vi "Read Value.vi"(8 "error in (no error)":errorcluster caption="entrée d'erreur (pas d'erreur)", 11 "DAQmxTaskDInput_Emulate en entrée":refnum<class "DAQmxTaskDInput_Emulate.lvclass">) -> (0 "error out":errorcluster caption="sortie d'erreur", 1 "Data":bool, 2 "Data string":string, 3 "DAQmxTaskDInput_Emulate en sortie":refnum<class "DAQmxTaskDInput_Emulate.lvclass">)   [LabVIEW 2015, in "DAQmxTaskDInput_Emulate.lvclass"]
uses:
  DAQmxTaskDInput_Emulate.lvclass
  DAQmxTaskDInput_Emulate.lvclass/DAQmxTaskDInput_Emulate.ctl
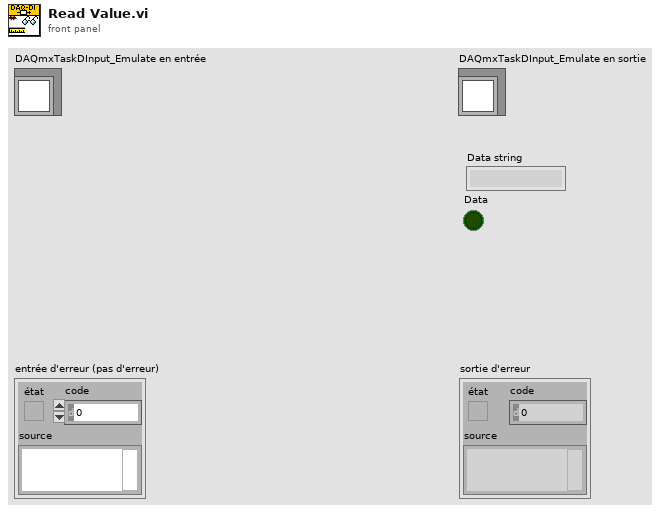
[diagram p1: front panel]
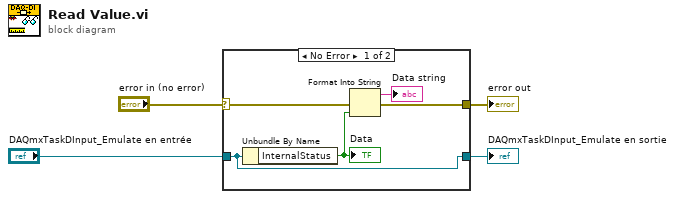
[diagram p0: block diagram]
diagram:
  n1 = case shown="No Error" "error in (no error)" {
    selector: "error in (no error)" -> [w9 w10]
    tunnel: [w8 w10] -> w3
    tunnel: "DAQmxTaskDInput_Emulate en entrée" -> [w5 w11]
    tunnel: [w5 w11] -> w1
    frame No Error {
      n2 = Unbundle By Name(w5) -> ("InternalStatus"=w6:bool)
      "Data" <- w6
      n3 = Format Into String(error in=w9, w6) -> (resulting string=→"Data string":string, error out=w8:errorcluster)  [unwired: 2 in]
    }
    frame Error {
    }
  }
  "error out" <- w3
  "DAQmxTaskDInput_Emulate en sortie" <- w1
